vi "FourFlippingCoins.vi"() -> ()   [LabVIEW 2014]
doc: "Problem Ch2 Do-It-Yourself\n\n This VI randomly determines the state of 4 'coins' in which they may either be heads or tails, for multiple iterations from which it produces a histogram. \n\nAt about 60 or more trials the results become more or less consistent with the statistically predicted values. Although there are numerous occasions when the distribution was completely wrong in which most trials where at 1 or 4 heads."
uses:
  <vilib>/Analysis/NI_AALBase.lvlib
panel:
  out "Waveform Graph":i32[](graph)
  out "Number of Heads":dbl
  in  "Total Number of Trials":dbl
  out "Coin 4":bool
  out "Coin 3":bool
  out "Coin 2":bool
  out "Coin 1":bool
  # "Heads = Lit"
  # "Tails =Unlit"
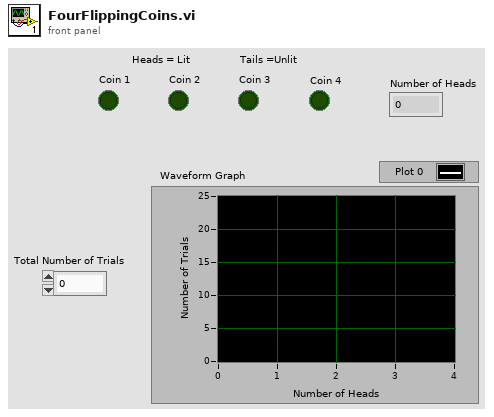
[diagram p1: front panel]
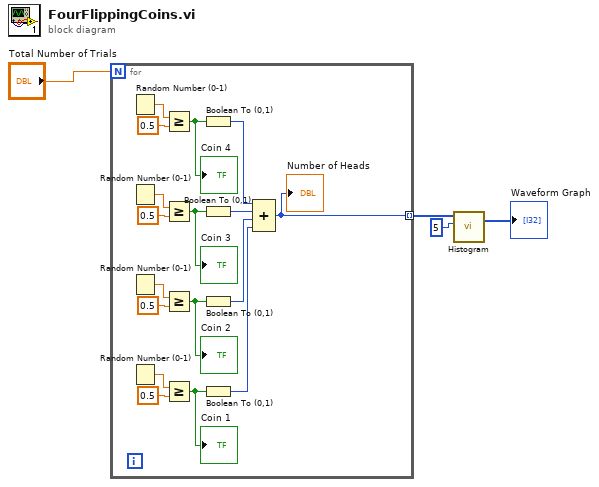
[diagram p0: block diagram]
diagram:
  n1 = for {
    N: "Total Number of Trials" -> [_]
    tunnel: [w5] -> w3 mode=indexing
    n2 = Random Number (0-1)() -> (number: 0 to 1=w15:dbl)
    n3 = Random Number (0-1)() -> (number: 0 to 1=w17:dbl)
    n4 = Random Number (0-1)() -> (number: 0 to 1=w19:dbl)
    n5 = Random Number (0-1)() -> (number: 0 to 1=w21:dbl)
    n6 = Greater Or Equal?(x=w15, y=0.5) -> (x >= y?=w7:bool)
    "Coin 4" <- w7
    n7 = Greater Or Equal?(x=w17, y=0.5) -> (x >= y?=w8:bool)
    "Coin 3" <- w8
    n8 = Greater Or Equal?(x=w19, y=0.5) -> (x >= y?=w9:bool)
    "Coin 2" <- w9
    n9 = Greater Or Equal?(x=w21, y=0.5) -> (x >= y?=w6:bool)
    "Coin 1" <- w6
    n10 = Boolean To (0,1)(Boolean=w7) -> (0, 1=w13:i16)
    n11 = Boolean To (0,1)(Boolean=w8) -> (0, 1=w12:i16)
    n12 = Boolean To (0,1)(Boolean=w9) -> (0, 1=w11:i16)
    n13 = Boolean To (0,1)(Boolean=w6) -> (0, 1=w10:i16)
    n14 = Compound Arithmetic op=ADD(w13, w12, w11, w10) -> (w5:i16)
    "Number of Heads" <- w5
  }
  n15 = call <vilib>:"Histogram.vi"("intervals"=5, "X"=w3) -> ("Histogram: h(x)"=→"Waveform Graph":i32[])  [unwired: 6 in, 3 out]
